vi "String 2 String Array.vi"(0 "String":string, 1 "Delimiter (\",\")":string=",") -> (2 "Substrings":string[](array[string]))   [LabVIEW 2016, in "CS++Utilities.lvlib"]
doc: "This VI converts a <b>String</b> of <b>Delimiter</b> separated substrings into an array of substrings."
uses:
  CS++Utilities.lvlib
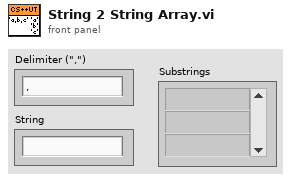
[diagram p1: front panel]
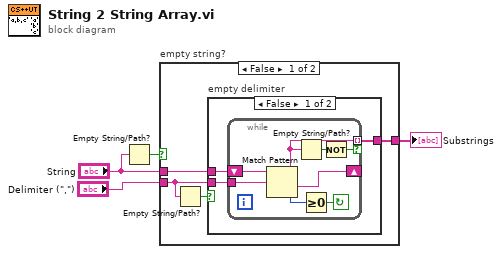
[diagram p0: block diagram]
diagram:
  n1 = Empty String/Path?(string/path="String") -> (empty?=w1:bool)
  n2 = case "empty string?" shown="False" w1 {
    tunnel: "Delimiter (\",\")" -> [w5 _]
    tunnel: [w8 _] -> w3
    tunnel: "String" -> [w7 _]
    frame False {
      n3 = Empty String/Path?(string/path=w5) -> (empty?=w6:bool)
      n4 = case "empty delimiter" shown="False" w6 {
        tunnel: w5 -> [w11 _]
        tunnel: [w10 _] -> w8
        tunnel: w7 -> [w9 _]
        frame False {
          n5 = while {
            shift-right: [w18] -> _
            shift-left: w9 -> [w19]
            tunnel: [w14] -> w10 mode=indexing if=w13
            tunnel: w11 -> [w12]
            stop <- w16 continue-if-true
            n6 = Match Pattern(string=w19, regular expression=w12) -> (before substring=w14:string, after substring=w18:string, offset past match=w17:i32)  [unwired: 1 in, 1 out]
            n7 = Empty String/Path?(string/path=w14) -> (empty?=w15:bool)
            n8 = Greater Or Equal To 0?(x=w17) -> (x >= 0?=w16:bool)
            n9 = Not(x=w15) -> (.not. x?=w13:bool)
          }
        }
        frame True {
        }
      }
    }
    frame True {
    }
  }
  "Substrings" <- w3
